vi "Main.Initialize.vi"(8 "error in (no error)":errorcluster, 10 "PCL":u32, 11 "Compiled Settings":T21 {"Nodes"."Monitor"."Network"."Name" format="%.0x"; "Nodes"."Sim"."Network"."Name" format="%.0x"; "XNET"."Termination" items=["Off", "On"]}) -> (0 "error out":errorcluster, 3 "State Variables":T1 {"Protocol"."Monitor.Network"."Name" format="%.0x"; "Protocol"."Data"."Trigger.Refs"."Data Reference" format="%.0x"; "Protocol"."Data"."Disable.Refs"."Data Reference" format="%.0x"; "Protocol"."Data"."Timing.Refs"."Data Reference" format="%.0x"; "Protocol"."Data"."Network"."Name" format="%.0x"; "Protocol"."Data"."Incoming.Refs"."Data Reference" format="%.0x"; "Protocol"."Data"."Outgoing.Refs"."Data Reference" format="%.0x"; "Protocol"."XNET.Settings"."Termination" items=["Off", "On"]})   [LabVIEW 2023, in "J1939 Addon Engine.lvlib"]
uses:
  J1939 Addon Engine.lvlib
  Addon Shared/Types/Compile Addon Settings.ctl
  Addon Shared/Types/XNET Settings.ctl
  Addon Shared/Types/SysDef FPGA Settings.ctl
  Addon Shared/Types/Compiled.Node Settings.ctl
  Addon Shared/Types/Compiled Monitor Tool Settings.ctl
  Addon Shared/Types/Monitor Settings.ctl
  Addon Shared/Types/Device Settings.ctl
  Addon Shared/Types/Incoming Settings.ctl
  Addon Shared/Types/Incoming Frame Settings.ctl
  <vilib>/NI VeriStand/Custom Device API/Block Data Reference.ctl
  <vilib>/NI VeriStand/Custom Device API/Data Reference.ctl
  Addon Shared/Types/Outgoing Settings.ctl
  Addon Shared/Types/Outgoing Frame Settings.ctl
  Addon Shared/Types/Outgoing Event Trigger Types.ctl
  SubModules/Frame-Protection-Support/Source/Shared/Types/Exported Frame Settings.ctl
  SubModules/Frame-Protection-Support/Source/Shared/Types/Exported Frame Type.ctl
  SubModules/Frame-Protection-Support/Source/Shared/Types/Exported Protection Settings.ctl
  SubModules/Frame-Protection-Support/Source/Shared/Types/Protection Type.ctl
  SubModules/Frame-Protection-Support/Source/Shared/Types/XNET Signal Configuration.ctl
  SubModules/Frame-Protection-Support/Source/Shared/Types/Exported Counter Settings.ctl
  SubModules/Frame-Protection-Support/Source/Shared/Types/Exported Event Trigger Type.ctl
  Addon Shared/Types/Complied Simulated Device Settings.ctl
  Addon Shared/Types/Compiled Simulated Settings.ctl
  Types/Main.State Variables.ctl
  <vilib>/NI/NIVS Inline Async API/_VS Inline Async API/VS Inline Async API/VS Inline Async API.lvclass
  Types/Main.Settings.ctl
  Types/Protocol.App Settings.ctl
  Types/Protocol.XNET Refs.ctl
  Types/Main.Outgoing.Frame.Settings.ctl
  Types/Engine.DTC Settings.ctl
  Types/Engine.DTC FIFOs.ctl
  <vilib>/NI VeriStand/Custom Device API/Custom Device API.lvlib
  Addon Shared/J1939 Addon Shared.lvlib
  SubModules/Frame-Protection-Support/Source/Shared/Protection and Counter Support Shared.lvlib
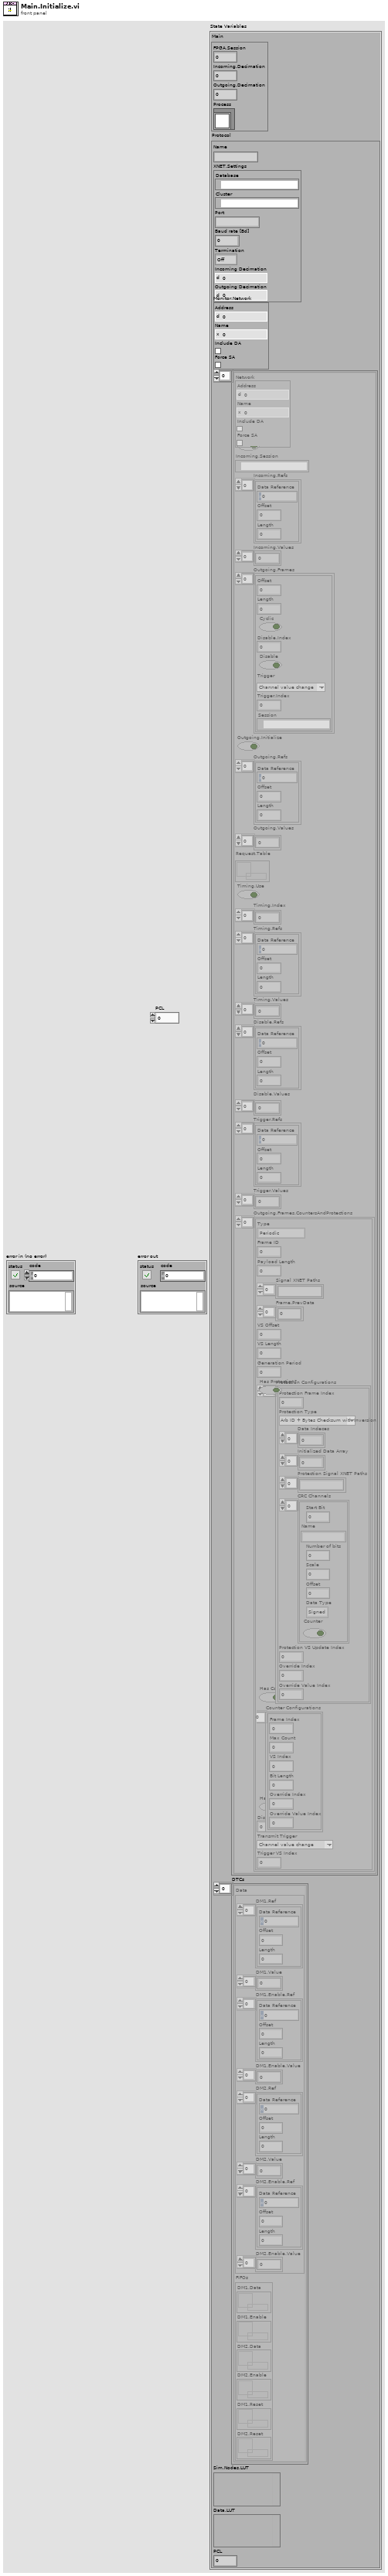
[diagram p1: front panel]
types:
  T1 = typedef "J1939 Addon Engine.lvlib/Main.State Variables.ctl" = cluster{"Main":T2, "Protocol":T3}
  T2 = typedef "J1939 Addon Engine.lvlib/Main.Settings.ctl" = cluster{"FPGA.Session":u32, "Incoming.Decimation":u32, "Outgoing.Decimation":u32, "Process":refnum<class "VS Inline Async API.lvclass">}
  T3 = typedef "J1939 Addon Engine.lvlib/Protocol.App Settings.ctl" = cluster{"Name":string, "XNET.Settings":T4, "Monitor.Network":T5, "Data":T6[], "DTCs":T18[], "Sim.Nodes.LUT":variant, "Data.LUT":variant, "PCL":u32}
  T4 = typedef "J1939 Addon Shared.lvlib/XNET Settings.ctl" = cluster{"Database":refnum<k21>, "Cluster":refnum<k21>, "Port":string, "Baud rate [Bd]":u32, "Termination":u32, "Incoming Decimation":u32, "Outgoing Decimation":u32}
  T5 = typedef "J1939 Addon Shared.lvlib/Monitor Settings.ctl" = cluster{"Address":u8, "Name":u64, "Include DA":bool, "Force SA":bool}
  T6 = typedef "J1939 Addon Engine.lvlib/Protocol.XNET Refs.ctl" = cluster{"Network":T5, "Incoming.Use":bool, "Incoming.Session":refnum<k21>, "Incoming.Refs":T7[], "Incoming.Values":dbl[], "Outgoing.Frames":T9[], "Outgoing.Initialize":bool, "Outgoing.Refs":T7[], "Outgoing.Values":dbl[], "Request.Table":refnum<k33>, "Timing.Use":bool, "Timing.Index":i32[], "Timing.Refs":T7[], "Timing.Values":dbl[], "Disable.Refs":T7[], "Disable.Values":dbl[], "Trigger.Refs":T7[], "Trigger.Values":dbl[], "Outgoing.Frames.CountersAndProtections":T11[]}
  T7 = typedef "Custom Device API.lvlib/Block Data Reference.ctl" = cluster{"Data Reference":T8, "Offset":u64, "Length":u64}
  T8 = typedef "Custom Device API.lvlib/Data Reference.ctl" = i32
  T9 = typedef "J1939 Addon Engine.lvlib/Main.Outgoing.Frame.Settings.ctl" = cluster{"Offset":u32, "Length":u32, "Cyclic":bool, "Disable.Index":i32, "Disable":bool, "Trigger":T10, "Trigger.Index":i32, "Session":refnum<k21>}
  T10 = typedef "J1939 Addon Shared.lvlib/Outgoing Event Trigger Types.ctl" = enum16{"Channel value change", "Trigger channel (not zero)", "Channel value change or trigger channel (not zero)", "Trigger channel (any value change)", "Channel value change or trigger channel (any value change)"}
  T11 = typedef "Protection and Counter Support Shared.lvlib/Exported Frame Settings.ctl" = cluster{"Type":T12, "Frame ID":u32, "Payload Length":u32, "Signal XNET Paths":string[], "Frame.PrevData":dbl[], "VS Offset":i32, "VS Length":i32, "Generation Period":u32, "Has Protection?":bool, "Protection Configurations":T13[], "Has Counter":bool, "Counter Configurations":T16[], "Has Disable?":bool, "Disable VS Index":i32, "Transmit Trigger":T17, "Trigger VS Index":i32}
  T12 = typedef "Protection and Counter Support Shared.lvlib/Exported Frame Type.ctl" = enum16{"Periodic", "Event", "Periodic/Event"}
  T13 = typedef "Protection and Counter Support Shared.lvlib/Exported Protection Settings.ctl" = cluster{"Protection Frame Index":i32, "Protection Type":T14, "Data Indeces":i32[], "Initialized Data Array":dbl[], "Protection Signal XNET Paths":string[], "CRC Channels":T15[], "Protection VS Update Index":i32, "Override Index":i32, "Override Value Index":i32}
  T14 = typedef "Protection and Counter Support Shared.lvlib/Protection Type.ctl" = enum16{"Arb ID + Bytes Checksum with Inversion", "Arb ID + Bytes CRC with Inversion", "Reversed Raw Signal Checksum with Inversion", "Concatenated Two's Compliment"}
  T15 = typedef "Protection and Counter Support Shared.lvlib/XNET Signal Configuration.ctl" = cluster{"Start Bit":i32, "Name":string, "Number of bits":i32, "Scale":dbl, "Offset":dbl, "Data Type":u32, "Counter":bool}
  T16 = typedef "Protection and Counter Support Shared.lvlib/Exported Counter Settings.ctl" = cluster{"Frame Index":i32, "Max Count":dbl, "VS Index":i32, "Bit Length":i64, "Override Index":i32, "Override Value Index":i32}
  T17 = typedef "Protection and Counter Support Shared.lvlib/Exported Event Trigger Type.ctl" = enum16{"Channel value change", "Trigger channel (not zero)", "Channel value change or trigger channel (not zero)", "Trigger channel (any value change)", "Channel value change or trigger channel (any value change)"}
  T18 = typedef "J1939 Addon Engine.lvlib/Engine.DTC Settings.ctl" = cluster{"Data":T19, "FIFOs":T20}
  T19 = typedef "J1939 Addon Shared.lvlib/Compiled Simulated Settings.ctl" = cluster{"DM1.Ref":T7[], "DM1.Value":dbl[], "DM1.Enable.Ref":T7[], "DM1.Enable.Value":dbl[], "DM2.Ref":T7[], "DM2.Value":dbl[], "DM2.Enable.Ref":T7[], "DM2.Enable.Value":dbl[]}
  T20 = typedef "J1939 Addon Engine.lvlib/Engine.DTC FIFOs.ctl" = cluster{"DM1.Data":refnum<k33>, "DM1.Enable":refnum<k33>, "DM2.Data":refnum<k33>, "DM2.Enable":refnum<k33>, "DM1.Reset":refnum<k33>, "DM2.Reset":refnum<k33>}
  T21 = typedef "J1939 Addon Shared.lvlib/Compile Addon Settings.ctl" = cluster{"XNET":T4, "Bitfile":T22, "Nodes":T23, "Name":string}
  T22 = typedef "J1939 Addon Shared.lvlib/SysDef FPGA Settings.ctl" = cluster{"RT Path":path, "RIO Device":string, "Enable":bool}
  T23 = typedef "J1939 Addon Shared.lvlib/Compiled.Node Settings.ctl" = cluster{"Monitor":T24, "Sim":T30[]}
  T24 = typedef "J1939 Addon Shared.lvlib/Compiled Monitor Tool Settings.ctl" = cluster{"Network":T5, "Data":T25}
  T25 = typedef "J1939 Addon Shared.lvlib/Device Settings.ctl" = cluster{"Incoming":T26, "Outgoing":T28}
  T26 = typedef "J1939 Addon Shared.lvlib/Incoming Settings.ctl" = cluster{"Signals":string[], "Frames":T27[], "Data.Refs":T7[], "Data.Values":dbl[], "Timing.Use":bool, "Timing.Refs":T7[], "Timing.Values":dbl[], "Timing.Index":i32[]}
  T27 = typedef "J1939 Addon Shared.lvlib/Incoming Frame Settings.ctl" = cluster{"Signals":string[], "PGN":u32}
  T28 = typedef "J1939 Addon Shared.lvlib/Outgoing Settings.ctl" = cluster{"Frames":T29[], "Data.Refs":T7[], "Data.Values":dbl[], "Disable.Refs":T7[], "Disable.Values":dbl[], "Trigger.Refs":T7[], "Trigger.Values":dbl[], "Frames.CountersAndProtections":T11[]}
  T29 = typedef "J1939 Addon Shared.lvlib/Outgoing Frame Settings.ctl" = cluster{"Signals":string[], "Channel Array Position":cluster{"Offset":u32, "Length":u32}, "PGN":u32, "Cyclic?":bool, "Disable?":bool, "Disable.Index":i32, "Trigger":T10, "Trigger.Index":i32}
  T30 = typedef "J1939 Addon Shared.lvlib/Complied Simulated Device Settings.ctl" = cluster{"Network":T5, "Data":T25, "DTCs":T19}
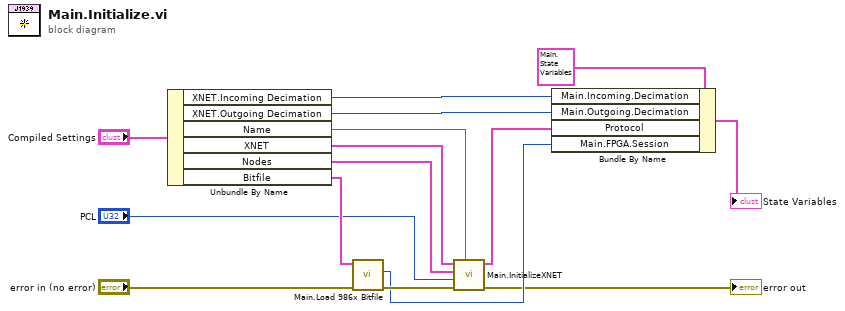
[diagram p0: block diagram]
diagram:
  n1 = Unbundle By Name("Compiled Settings") -> ("XNET.Incoming Decimation"=w14:u32, "XNET.Outgoing Decimation"=w15:u32, "Name"=w2:string, "XNET"=w8:T4, "Nodes"=w9:T23, "Bitfile"=w6:T22)
  n2 = call "Main.Load 986x Bitfile.vi"("error in (no error)"="error in (no error)", "FPGA Settings"=w6) -> ("error out"=w7:errorcluster, "FPGA Session"=w5:u32)  [unwired: 8 in]
  n3 = call "Main.InitializeXNET.vi"("Name"=w2, "error in (no error)"=w7, "PCL"="PCL", "Data Settings"=w9, "XNET Settings"=w8) -> ("error out"=→"error out":errorcluster, "Protocol App"=w4:T3)  [unwired: 5 in]
  n4 = Bundle By Name(cluster=T1 {"Main"={"FPGA.Session"=0, "Incoming.Decimation"=0, "Outgoing.Decimation"=0, "Process"=refnum}, "Protocol"={"Name"="", "XNET.Settings"={"Database"="", "Cluster"="", "Port"="", "Baud rate [Bd]"=0, "Termination"=0, "Incoming Decimation"=0, "Outgoing Decimation"=0}, "Monitor.Network"={"Address"=0, "Name"=0, "Include DA"=FALSE, "Force SA"=FALSE}, "Data"=[], "DTCs"=[], "Sim.Nodes.LUT"=variant, "Data.LUT"=variant, "PCL"=0}}, "Main.Incoming.Decimation"=w14, "Main.Outgoing.Decimation"=w15, "Protocol"=w4, "Main.FPGA.Session"=w5) -> (→"State Variables":T1)
